vi "Write config.vi"(8 "error in (no error)":errorcluster, 10 "FCR config params":T1={"VISA resource"="", "baud rate"=9600, "Acceleration"=0.0, "Velocity"=0.0, "Initial P1"=0.0, "Initial P2"=0.0}, 11 "DAQ config params":T2={"DAQ Device Name"="Dev2", "Physical channel"=""}) -> (0 "error out":errorcluster)   [LabVIEW 2020]
uses:
  controls/DAQ config parameters -- cluster.ctl
  controls/FCR config parameters -- cluster.ctl
  <vilib>/Utility/config.llb/Write Key (String).vi
  <vilib>/Utility/config.llb/Write Key (U32).vi
  <vilib>/Utility/config.llb/Write Key (Double).vi
  <vilib>/Utility/config.llb/NI_LVConfig.lvlib
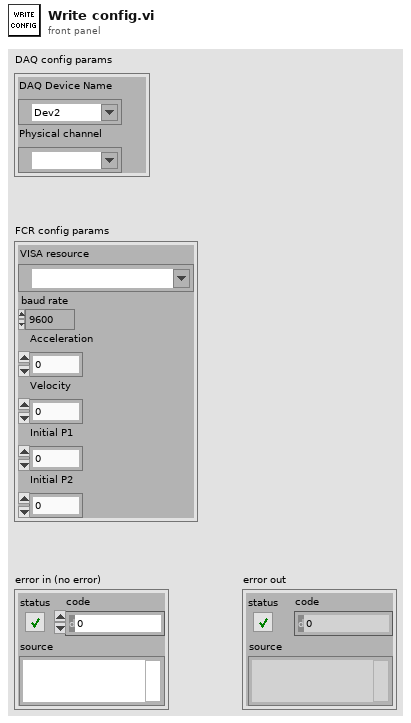
[diagram p1: front panel]
types:
  T1 = typedef "FCR config parameters -- cluster.ctl" = cluster{"VISA resource":refnum<visa-resource-name>, "baud rate":u32, "Acceleration":dbl, "Velocity":dbl, "Initial P1":dbl, "Initial P2":dbl}
  T2 = typedef "DAQ config parameters -- cluster.ctl" = cluster{"DAQ Device Name":tag, "Physical channel":tag}
  T3 = typedef "NI_LVConfig.lvlib/Config Data RefNum.ctl" = refnum<k1>
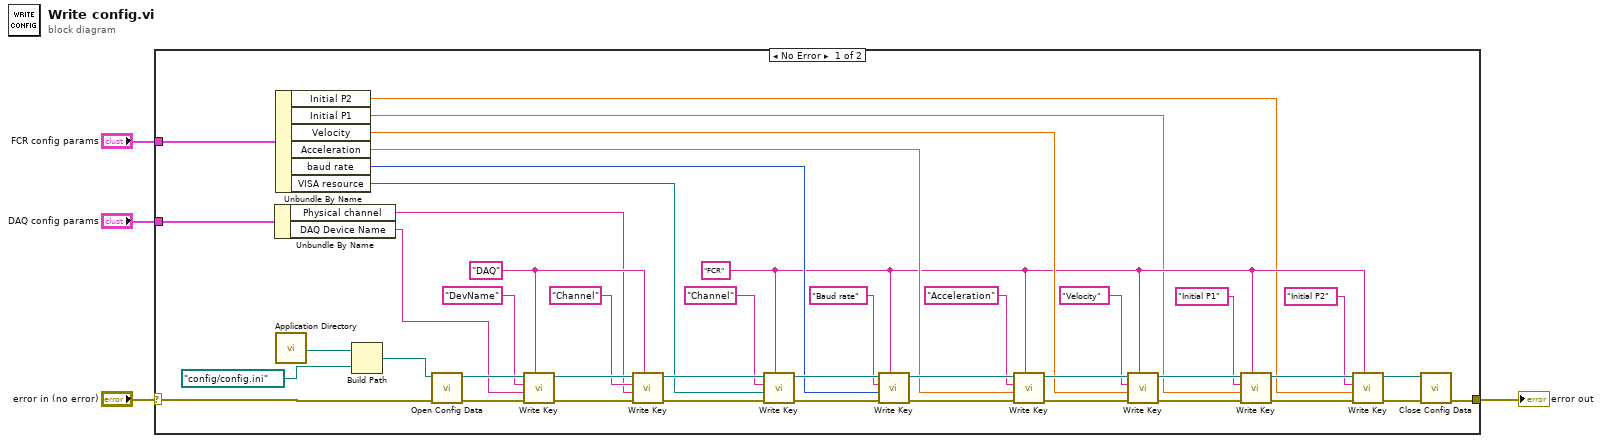
[diagram p0: block diagram]
diagram:
  n1 = case shown="No Error" "error in (no error)" {
    selector: "error in (no error)" -> [w44 w48]
    tunnel: "DAQ config params" -> [w42 _]
    tunnel: [w35 w48] -> w2
    tunnel: "FCR config params" -> [w32 _]
    frame No Error {
      w8 = "FCR" ("section")
      w36 = "DAQ" ("section")
      n2 = Unbundle By Name(w42) -> ("Physical channel"=w33:tag, "DAQ Device Name"=w39:tag)
      n3 = Unbundle By Name(w32) -> ("Initial P2"=w5:dbl, "Initial P1"=w6:dbl, "Velocity"=w17:dbl, "Acceleration"=w19:dbl, "baud rate"=w24:u32, "VISA resource"=w29:refnum<visa-resource-name>)
      n4 = call <vilib>:"Application Directory.vi"() -> ("Application Directory"=w47:path)
      n5 = Build Path(base path=w47, name or relative path=path "config/config.ini") -> (appended path=w45:path)
      n6 = call <vilib>:"Open Config Data.vi"("error in (no error)"=w44, "configuration file path"=w45) -> ("error out"=w43:errorcluster, "refnum"=w41:T3)  [unwired: 7 in, 1 out]
      n7 = call-poly <vilib>:"Write Key.vi"("section"=w36, "error in (no error)"=w43, "value"=w39, "key"="DevName", "refnum"=w41) -> ("error out"=w38:errorcluster, "refnum out"=w37:T3)  [unwired: 4 in, 1 out]
      n8 = call-poly <vilib>:"Write Key.vi"("section"=w36, "error in (no error)"=w38, "value"=w33, "key"="Channel", "refnum"=w37) -> ("error out"=w31:errorcluster, "refnum out"=w30:T3)  [unwired: 4 in, 1 out]
      n9 = call-poly <vilib>:"Write Key.vi"("section"=w8, "error in (no error)"=w31, "value"=w29, "key"="Channel", "refnum"=w30) -> ("error out"=w27:errorcluster, "refnum out"=w26:T3)  [unwired: 4 in, 1 out]
      n10 = call-poly <vilib>:"Write Key.vi"("section"=w8, "error in (no error)"=w27, "value"=w24, "key"="Baud rate", "refnum"=w26) -> ("error out"=w23:errorcluster, "refnum out"=w22:T3)  [unwired: 4 in, 1 out]
      n11 = call-poly <vilib>:"Write Key.vi"("section"=w8, "error in (no error)"=w23, "value"=w19, "key"="Acceleration", "refnum"=w22) -> ("error out"=w21:errorcluster, "refnum out"=w20:T3)  [unwired: 4 in, 1 out]
      n12 = call-poly <vilib>:"Write Key.vi"("section"=w8, "error in (no error)"=w21, "value"=w17, "key"="Velocity", "refnum"=w20) -> ("error out"=w15:errorcluster, "refnum out"=w14:T3)  [unwired: 4 in, 1 out]
      n13 = call-poly <vilib>:"Write Key.vi"("section"=w8, "error in (no error)"=w15, "value"=w6, "key"="Initial P1", "refnum"=w14) -> ("error out"=w12:errorcluster, "refnum out"=w10:T3)  [unwired: 4 in, 1 out]
      n14 = call-poly <vilib>:"Write Key.vi"("section"=w8, "error in (no error)"=w12, "value"=w5, "key"="Initial P2", "refnum"=w10) -> ("error out"=w11:errorcluster, "refnum out"=w9:T3)  [unwired: 4 in, 1 out]
      n15 = call <vilib>:"Close Config Data.vi"("error in (no error)"=w11, "refnum"=w9) -> ("error out"=w35:errorcluster)  [unwired: 8 in, 1 out]
    }
    frame Error {
    }
  }
  "error out" <- w2
